vi "Get Timing Data.vi"(2 "Previous Timing Data":i32[](array[numeric]), 3 "Previous Tick Count":u32) -> (0 "Timing Data":i32[](array[numeric]), 1 "Tick Count":u32)   [LabVIEW 2011, in "LabVIEW Interface for Arduino.lvlib"]
doc: "Record timing data in a while loop for use with Calculate Update Rates VI."
uses:
  LabVIEW Interface for Arduino.lvlib
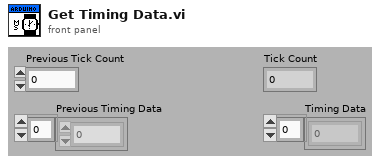
[diagram p1: front panel]
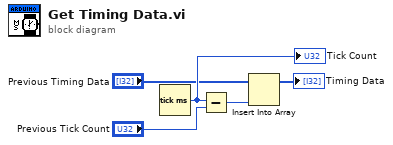
[diagram p0: block diagram]
diagram:
  n1 = Tick Count (ms)() -> (millisecond timer value=w5:u32)
  "Tick Count" <- w5
  n2 = Subtract(x=w5, y="Previous Tick Count") -> (x-y=w1:u32)
  n3 = Insert Into Array(array="Previous Timing Data", new element=w1) -> (→"Timing Data":i32[])  [unwired: 1 in]
